vi "Mutate Device Driver Path.vi"(8 "error in (no error)":errorcluster, 10 "Version":string="2020.0.0.0", 11 "Device Ref in":T1 format="%.0x") -> (0 "error out":errorcluster, 3 "Device Ref out":T1 format="%.0x")   [LabVIEW 2027, in "Embedded Data Logger System Explorer.lvlib"]
uses:
  Embedded Data Logger System Explorer.lvlib
  C:/NetCore/niveristand-embedded-data-logger-custom-device/Source/System Explorer/Mutate Device Driver Path.vi/NationalInstruments.VeriStand.SystemDefinitionAPI
  NationalInstruments.VeriStand.SystemDefinitionAPI
  <vilib>/NI VeriStand/Custom Device API/Path Type.ctl
  <vilib>/NI VeriStand/Custom Device API/Custom Device API.lvlib
  <vilib>/NI VeriStand/Custom Device API/Path Specification.ctl
  <vilib>/NI VeriStand/Custom Device API/Custom Device Supported Target.ctl
  <vilib>/NI VeriStand/Custom Device API/Custom Device Path Data.ctl
  <vilib>/NI VeriStand/Custom Device API/Custom Device Item Ref.ctl
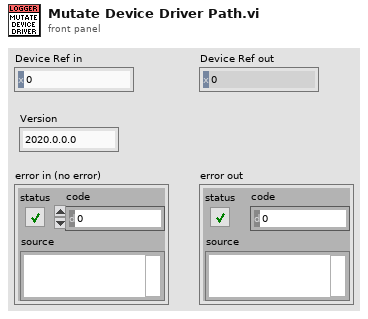
[diagram p1: front panel]
types:
  T1 = typedef "Custom Device API.lvlib/Custom Device Item Ref.ctl" = u64
  T2 = typedef "Custom Device API.lvlib/Custom Device Path Data.ctl" = cluster{"SupportedTarget":T3, "Source":T4, "RT Destination":path}
  T3 = typedef "Custom Device API.lvlib/Custom Device Supported Target.ctl" = enum16{"All", "PharLap", "VxWorks", "Windows", "Linux_32_ARM", "Linux_x64", "PharLap & Windows", "PharLap & VxWorks", "VxWorks & Windows"}
  T4 = typedef "Custom Device API.lvlib/Path Specification.ctl" = cluster{"Path":path, "Type":T5}
  T5 = typedef "Custom Device API.lvlib/Path Type.ctl" = enum16{"Absolute", "To Base", "To Common Data Dir", "To Application Data Dir"}
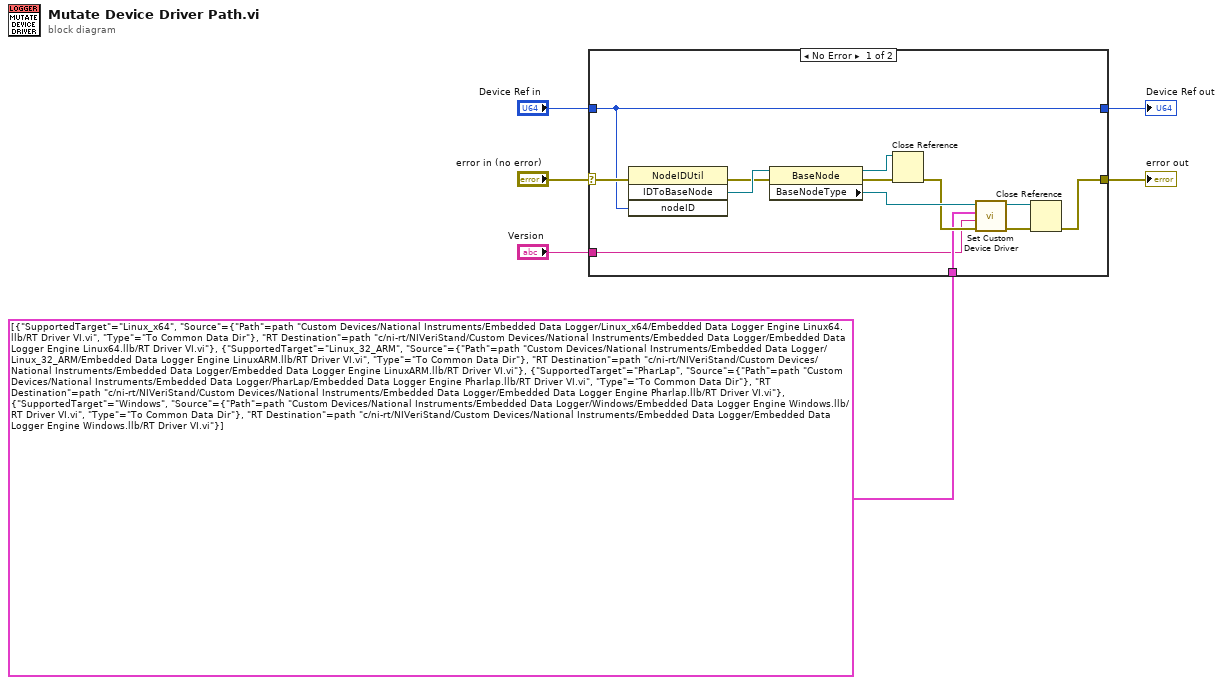
[diagram p0: block diagram]
diagram:
  n1 = case shown="No Error" "error in (no error)" {
    selector: "error in (no error)" -> [w15 w21]
    tunnel: [w9 w21] -> w5
    tunnel: "Device Ref in" -> [w12 w20]
    tunnel: [w12 w20] -> w3
    tunnel: T2[] [{"SupportedTarget"=enum."Linux_x64", "Source"={"Path"=path "Custom Devices/National Instruments/Embedded Data Logger/Linux_x64/Embedded Data Logger Engine Linux64.llb/RT Driver VI.vi", "Type"=enum."To Common Data Dir"}, "RT Destination"=path "c:/ni-rt/NIVeriStand/Custom Devices/National Instruments/Embedded Data Logger/Embedded Data Logger Engine Linux64.llb/RT Driver VI.vi"}, {"SupportedTarget"=enum."Linux_32_ARM", "Source"={"Path"=path "Custom Devices/National Instruments/Embedded Data Logger/Linux_32_ARM/Embedded Data Logger Engine LinuxARM.llb/RT Driver VI.vi", "Type"=enum."To Common Data Dir"}, "RT Destination"=path "c:/ni-rt/NIVeriStand/Custom Devices/National Instruments/Embedded Data Logger/Embedded Data Logger Engine LinuxARM.llb/RT Driver VI.vi"}, {"SupportedTarget"=enum."PharLap", "Source"={"Path"=path "Custom Devices/National Instruments/Embedded Data Logger/PharLap/Embedded Data Logger Engine Pharlap.llb/RT Driver VI.vi", "Type"=enum."To Common Data Dir"}, "RT Destination"=path "c:/ni-rt/NIVeriStand/Custom Devices/National Instruments/Embedded Data Logger/Embedded Data Logger Engine Pharlap.llb/RT Driver VI.vi"}, {"SupportedTarget"=enum."Windows", "Source"={"Path"=path "Custom Devices/National Instruments/Embedded Data Logger/Windows/Embedded Data Logger Engine Windows.llb/RT Driver VI.vi", "Type"=enum."To Common Data Dir"}, "RT Destination"=path "c:/ni-rt/NIVeriStand/Custom Devices/National Instruments/Embedded Data Logger/Embedded Data Logger Engine Windows.llb/RT Driver VI.vi"}] ("Driver VIs") -> [w8 _]
    tunnel: "Version" -> [w7 _]
    frame No Error {
      n2 = invoke class="NodeIDUtil" method="IDToBaseNode"(error in=w15, "nodeID"=w12) -> (error out=w16:errorcluster, "IDToBaseNode"=w17:refnum<k39>)  [unwired: 2 in, 2 out]
      n3 = property class="BaseNode"(reference=w17, error in=w16) -> (reference out=w18:refnum<k39>, error out=w19:errorcluster, "BaseNodeType"=w14:refnum<k39>)
      n4 = Close Reference(reference=w18, error in (no error)=w19) -> (error out=w13:errorcluster)
      n5 = call "Set Custom Device Driver.vi"("error in (no error)"=w13, "Version"=w7, "Driver VIs"=w8, "NationalInstruments.VeriStand.SystemStorage.BaseNodeType"=w14) -> ("error out"=w11:errorcluster, "NationalInstruments.VeriStand.SystemStorage.BaseNodeType"=w10:refnum<k39>)  [unwired: 6 in]
      n6 = Close Reference(reference=w10, error in (no error)=w11) -> (error out=w9:errorcluster)
    }
    frame Error {
    }
  }
  "error out" <- w5
  "Device Ref out" <- w3
